vi "Autonomous Independent.vi"() -> ()   [LabVIEW 2016]
doc: "This VI is called when autonomous begins, and will automatically be terminated when autonomous ends. You can carry out timed or sensor driven robot movement independently without needing to return to the caller."
uses:
  <vilib>/Rock Robotics/WPI/Utilities/WPI_GetSetVariantRefNum.vi
  <vilib>/Rock Robotics/Network Tables/NT Read String.vi
  Robot Global Data.vi
  <vilib>/Rock Robotics/Network Tables/NT Write Numeric Array.vi
panel:
  in  "stop distance":dbl
  in  "min drive speed":dbl
  in  "max drive speed":dbl
  in  "drive gain":dbl
  in  "turn gain":dbl
  out "right motor":dbl
  out "left motor":dbl
  out "center x 2":dbl
  out "center y 2":dbl
  out "turn speed":dbl
  in  "turn offset":dbl
  in  "setpoint":dbl
  out "motor speed":dbl
  out "center y":dbl
  out "center x":dbl
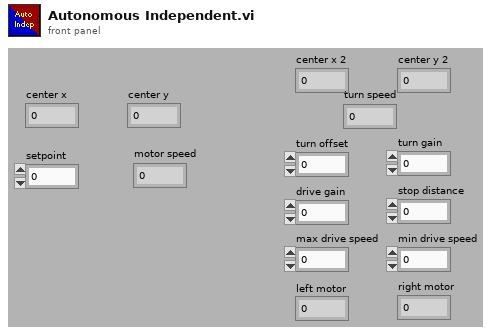
[diagram p1: front panel]
types:
  T1 = typedef "WPI_JoystickDevRef.ctl" = cluster{"Device":T2}
  T2 = typedef "WPI_JoystickDeviceEnum.ctl" = enum16{"USB 0", "USB 1", "USB 2", "USB 3", "USB 4", "USB 5"}
  T3 = cluster{"Distance (ft)":dbl, "Score":dbl, "Normalized":cluster{"Center":cluster{dbl, dbl}, "Rectangle":cluster{"Numeric":dbl, "Numeric 2":dbl, "Numeric 3":dbl, "Numeric 5":dbl}}, "Pixels":cluster{"Center":cluster{dbl, dbl}, "Rectangle":cluster{"Numeric":dbl, "Numeric 2":dbl, "Numeric 3":dbl, "Numeric 5":dbl}}}
  T4 = typedef "WPI_RobotDriveDevRef.ctl" = cluster{"DevStatus":errorcluster, "Motors[]":T5[], "Square Inputs":bool, "Max Output":dbl}
  T5 = typedef "WPI_MotorControlDeviceRef.ctl" = cluster{"DeviceStatus":errorcluster, "Type":T6, "PWM":cluster{"PWM Channel":T7, "DeadBand":T8}, "CAN":cluster{"Device Number":u8, "SetOutput VI Ref":variant, "GetOutput VI Ref":variant, "Enable VI Ref":variant, "Disable VI Ref":variant, "Data":variant}, "Invert":bool}
  T6 = typedef "WPI_MotorControlType.ctl" = enum16{"PWM", "CAN"}
  T7 = typedef "FPGA_DIOPWMChannel.ctl" = enum8{"PWM 0", "PWM 1", "PWM 2", "PWM 3", "PWM 4", "PWM 5", "PWM 6", "PWM 7", "PWM 8", "PWM 9", "PWM MXP 0", "PWM MXP 1", "PWM MXP 2", "PWM MXP 3", "PWM MXP 4", "PWM MXP 5", "PWM MXP 6", "PWM MXP 7", "PWM MXP 8", "PWM MXP 9", "Invalid"}
  T8 = typedef "WPI_PWMDeadband.ctl" = cluster{"Name":string, "maxPositivePwm":i32, "minPositivePwm":i32, "centerPwm":i32, "maxNegativePwm":i32, "minNegativePwm":i32, "angularRange":u16}
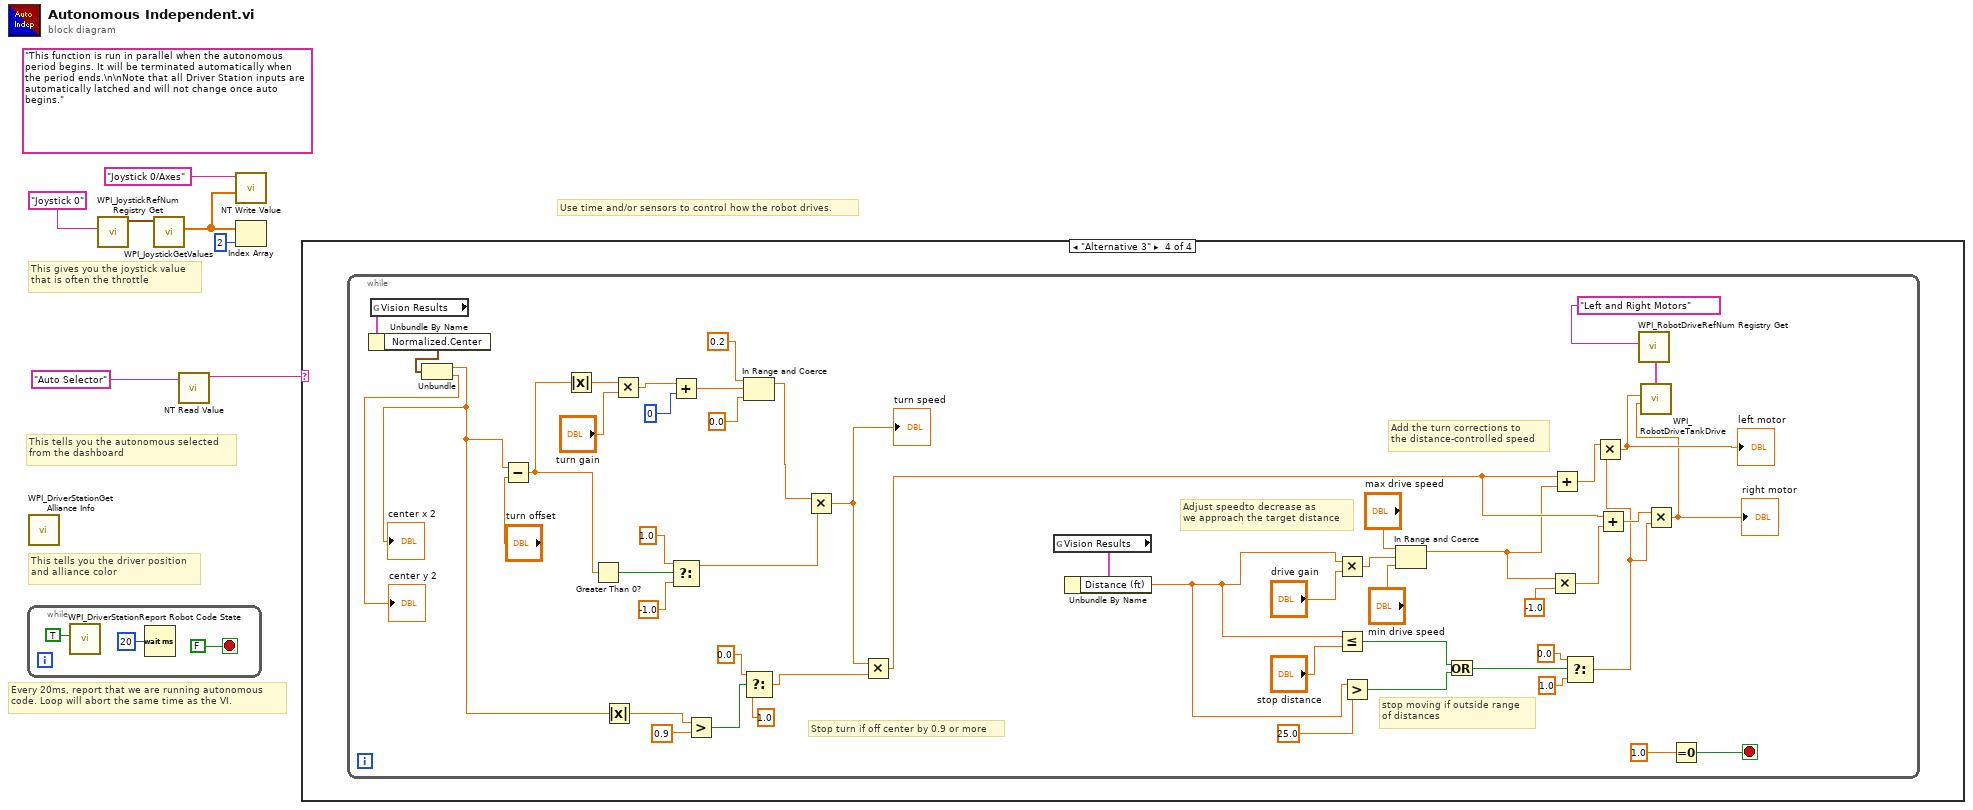
[diagram p0: block diagram]
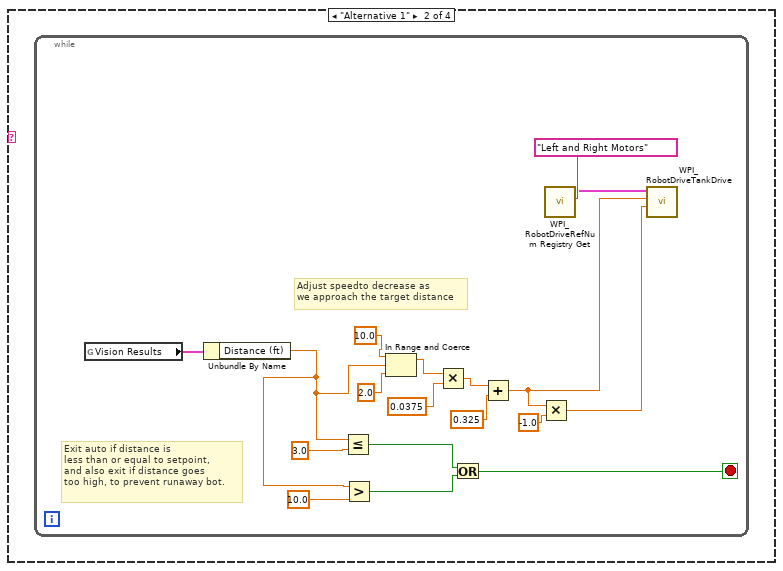
[diagram p3: hidden frame]
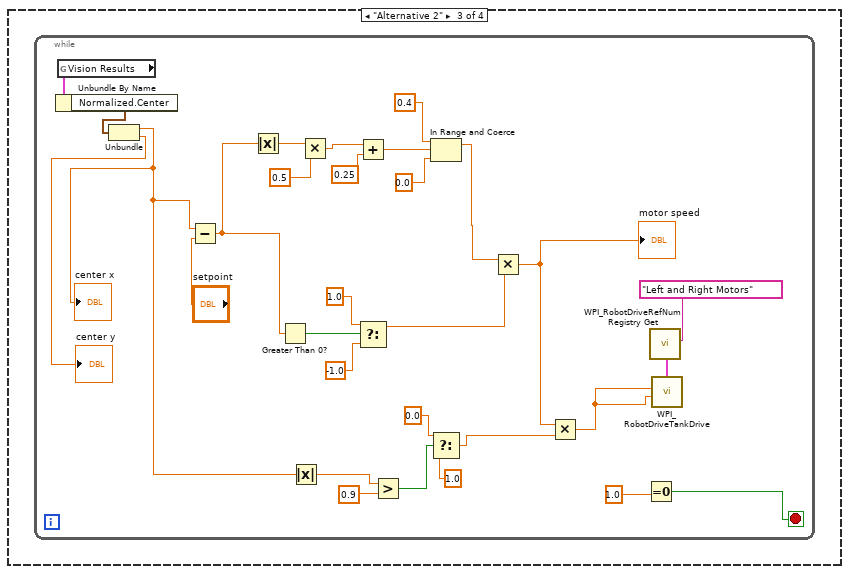
[diagram p4: hidden frame]
diagram:
  (unwired) "This function is run in parallel when the autonomous period begins. It will be terminated automatically when the period ends.\n\nNote that all Driver Station inputs are automatically latched and will not change once auto begins."
  # "This tells you the autonomous selected\nfrom the dashboard"
  # "Every 20ms, report that we are running autonomous\ncode. Loop will abort the same time as the VI."
  # "This gives you the joystick value\nthat is often the throttle"
  # "Use time and/or sensors to control how the robot drives."
  # "This tells you the driver position\nand alliance color"
  n1 = while {
    stop <- FALSE stop-if-true
    n2 = call <vilib>:"WPI_DriverStationReport Robot Code State.vi"("Autonomous"=TRUE) -> ()  [unwired: 10 in, 1 out]
    n3 = Wait (ms)(milliseconds to wait=u32 20) -> ()  [unwired: 1 out]
  }
  n4 = call <vilib>:"WPI_DriverStationGet Alliance Info.vi"() -> ()  [unwired: 12 out]
  n5 = call <vilib>:"WPI_JoystickRefNum Registry Get.vi"("refnum name"="Joystick 0") -> ("JoystickDevRef"=w6:T1)  [unwired: 1 in, 9 out]
  n6 = call <vilib>:"WPI_JoystickGetValues.vi"("JoystickDevRef"=w6) -> ("Axes"=w2:dbl[])  [unwired: 6 in, 4 out]
  n7 = call-poly <vilib>:"NT Read Value.vi"("Name"="Auto Selector") -> ("String"=w3:string)  [unwired: 9 in, 1 out]
  n8 = call-poly <vilib>:"NT Write Value.vi"("Numeric Array"=w2, "Name"="Joystick 0/Axes") -> ()  [unwired: 9 in, 1 out]
  n9 = Index Array(array=w2, index=2) -> ()  [unwired: 1 out]
  n10 = case shown="\"Alternative 3\"" w3 {
    frame Default {
      # "You can put your main auto here, or you can right-click on the case and make any\nother frame be the default case."
      # "This is the frame that will execute if no selection is made, or if it is not recognized"
    }
    frame "Alternative 1" {
      n11 = while {
        stop <- w11 stop-if-true
        # "Adjust speedto decrease as \nwe approach the target distance"
        # "Exit auto if distance is\nless than or equal to setpoint,\nand also exit if distance goes \ntoo high, to prevent runaway bot."
        n12 = global read "Robot Global Data.vi" "Vision Results"() -> (w28:T3)
        n13 = Unbundle By Name(w28) -> ("Distance (ft)"=w15:dbl)
        n14 = Less Or Equal?(x=w15, y=3.0) -> (x <= y?=w13:bool)
        n15 = Greater?(x=w15, y=10.0) -> (0:w12:bool)
        n16 = In Range and Coerce(upper limit=10.0 ("y"), x=w15, lower limit=2.0 ("y")) -> (coerced(x)=w22:dbl)  [unwired: 1 out]
        n17 = Multiply(x=w22, y=0.0375) -> (x*y=w20:dbl)
        n18 = Or(x=w13, y=w12) -> (x .or. y?=w11:bool)
        n19 = Add(x=w20, y=0.325) -> (x+y=w18:dbl)
        n20 = Multiply(x=w18, y=-1.0) -> (x*y=w16:dbl)
        n21 = call <vilib>:"WPI_RobotDriveRefNum Registry Get.vi"("refnum name"="Left and Right Motors") -> ("RobotDriveDevRef"=w26:T4)  [unwired: 9 in, 1 out]
        n22 = call <vilib>:"WPI_RobotDriveTankDrive.vi"("Right axis value"=w16, "Left axis value"=w18, "RobotDriveDevRef"=w26) -> ()  [unwired: 6 in, 3 out]
      }
    }
    frame "Alternative 2" {
      n23 = while {
        stop <- w32 stop-if-true
        n24 = global read "Robot Global Data.vi" "Vision Results"() -> (w58:T3)
        n25 = Unbundle By Name(w58) -> ("Normalized.Center"=w54:cluster{dbl, dbl})
        n26 = Unbundle(w54) -> (w30:dbl, →"center y":dbl)
        "center x" <- w30
        n27 = Subtract(x=w30, y="setpoint") -> (x-y=w29:dbl)
        n28 = Absolute Value(x=w29) -> (abs(x)=w46:dbl)
        n29 = Greater Than 0?(x=w29) -> (x > 0?=w51:bool)
        n30 = Absolute Value(x=w30) -> (abs(x)=w53:dbl)
        n31 = Multiply(x=w46, y=0.5) -> (x*y=w44:dbl)
        n32 = Add(x=w44, y=0.25) -> (x+y=w42:dbl)
        n33 = Select(t=1.0, s=w51, f=-1.0 ("t")) -> (s? t:f=w48:dbl)
        n34 = Greater?(x=w53, y=0.9) -> (0:w39:bool)
        n35 = In Range and Coerce(upper limit=0.4, x=w42, lower limit=0.0) -> (coerced(x)=w40:dbl)  [unwired: 1 out]
        n36 = Select(t=0.0, s=w39, f=1.0 ("t")) -> (s? t:f=w36:dbl)
        n37 = Multiply(x=w40, y=w48) -> (x*y=w35:dbl)
        "motor speed" <- w35
        n38 = Multiply(x=w35, y=w36) -> (x*y=w34:dbl)
        n39 = Equal To 0?(x=1.0 ("t")) -> (x = 0?=w32:bool)
        n40 = call <vilib>:"WPI_RobotDriveRefNum Registry Get.vi"("refnum name"="Left and Right Motors") -> ("RobotDriveDevRef"=w55:T4)  [unwired: 9 in, 1 out]
        n41 = call <vilib>:"WPI_RobotDriveTankDrive.vi"("Right axis value"=w34, "Left axis value"=w34, "RobotDriveDevRef"=w55) -> ()  [unwired: 6 in, 3 out]
      }
    }
    frame "Alternative 3" {
      n42 = while {
        stop <- w69 stop-if-true
        # "stop moving if outside range\nof distances"
        # "Stop turn if off center by 0.9 or more"
        # "Add the turn corrections to \nthe distance-controlled speed"
        # "Adjust speedto decrease as \nwe approach the target distance"
        n43 = global read "Robot Global Data.vi" "Vision Results"() -> (w109:T3)
        n44 = Unbundle By Name(w109) -> ("Normalized.Center"=w107:cluster{dbl, dbl})
        n45 = Unbundle(w107) -> (w87:dbl, →"center y 2":dbl)
        "center x 2" <- w87
        n46 = Subtract(x=w87, y="turn offset") -> (x-y=w86:dbl)
        n47 = Absolute Value(x=w86) -> (abs(x)=w99:dbl)
        n48 = Greater Than 0?(x=w86) -> (x > 0?=w104:bool)
        n49 = Absolute Value(x=w87) -> (abs(x)=w106:dbl)
        n50 = Multiply(x=w99, y="turn gain") -> (x*y=w98:dbl)
        n51 = Add(x=w98, y=0) -> (x+y=w96:dbl)
        n52 = Select(t=1.0, s=w104, f=-1.0 ("t")) -> (s? t:f=w101:dbl)
        n53 = Greater?(x=w106, y=0.9) -> (0:w93:bool)
        n54 = In Range and Coerce(upper limit=0.2, x=w96, lower limit=0.0) -> (coerced(x)=w94:dbl)  [unwired: 1 out]
        n55 = Select(t=0.0, s=w93, f=1.0 ("t")) -> (s? t:f=w90:dbl)
        n56 = Multiply(x=w94, y=w101) -> (x*y=w89:dbl)
        "turn speed" <- w89
        n57 = Multiply(x=w89, y=w90) -> (x*y=w78:dbl)
        n58 = global read "Robot Global Data.vi" "Vision Results"() -> (w85:T3)
        n59 = Unbundle By Name(w85) -> ("Distance (ft)"=w64:dbl)
        n60 = Multiply(x=w64, y="drive gain") -> (x*y=w63:dbl)
        n61 = Less Or Equal?(x=w64, y="stop distance") -> (x <= y?=w80:bool)
        n62 = Greater?(x=w64, y=25.0) -> (0:w79:bool)
        n63 = In Range and Coerce(upper limit="max drive speed", x=w63, lower limit="min drive speed") -> (coerced(x)=w60:dbl)  [unwired: 1 out]
        n64 = Or(x=w80, y=w79) -> (x .or. y?=w76:bool)
        n65 = Multiply(x=w60, y=-1.0) -> (x*y=w77:dbl)
        n66 = Add(x=w78, y=w60) -> (x+y=w73:dbl)
        n67 = Select(t=0.0, s=w76, f=1.0 ("t")) -> (s? t:f=w71:dbl)
        n68 = Multiply(x=w73, y=w71) -> (x*y=w68:dbl)
        "left motor" <- w68
        n69 = Add(x=w78, y=w77) -> (x+y=w72:dbl)
        n70 = call <vilib>:"WPI_RobotDriveRefNum Registry Get.vi"("refnum name"="Left and Right Motors") -> ("RobotDriveDevRef"=w83:T4)  [unwired: 9 in, 1 out]
        n71 = Multiply(x=w72, y=w71) -> (x*y=w67:dbl)
        "right motor" <- w67
        n72 = call <vilib>:"WPI_RobotDriveTankDrive.vi"("Right axis value"=w67, "Left axis value"=w68, "RobotDriveDevRef"=w83) -> ()  [unwired: 6 in, 3 out]
        n73 = Equal To 0?(x=1.0 ("t")) -> (x = 0?=w69:bool)
      }
    }
  }
